vi "ingresaMediciones.vi"(8 "error in (no error)":errorcluster, 9 "Tbl Refnum":refnum<vi>, 10 "New Value":string[][](array[string]), 11 "Prueba06 in":refnum<class "Prueba06.lvclass">) -> (0 "error out":errorcluster, 3 "Prueba06 out":refnum<class "Prueba06.lvclass">)   [LabVIEW 2019, in "Prueba06.lvclass"]
uses:
  Prueba06.lvclass
  Prueba06.lvclass/Prueba06.ctl
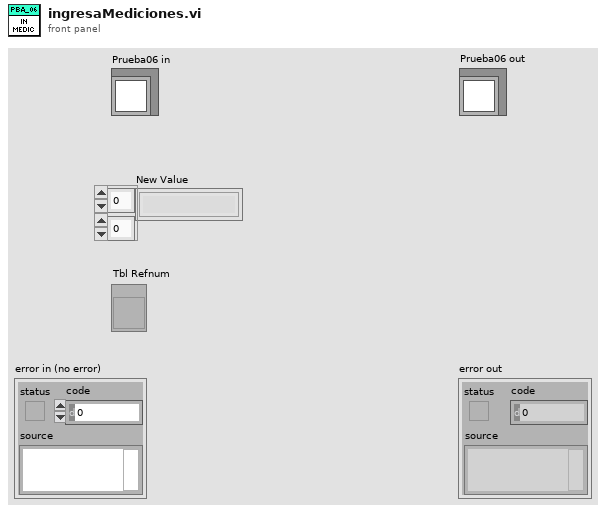
[diagram p1: front panel]
types:
  T1 = cluster{"Medido":dbl, "Error":dbl, "Ref":dbl, "Incert_exp":dbl, "Tol+":dbl, "Tol-":dbl, "fila":i32}
  T2 = typedef "LVRowAndColumnTypeDef.ctl" = cluster{"Row":i32, "Column":i32}
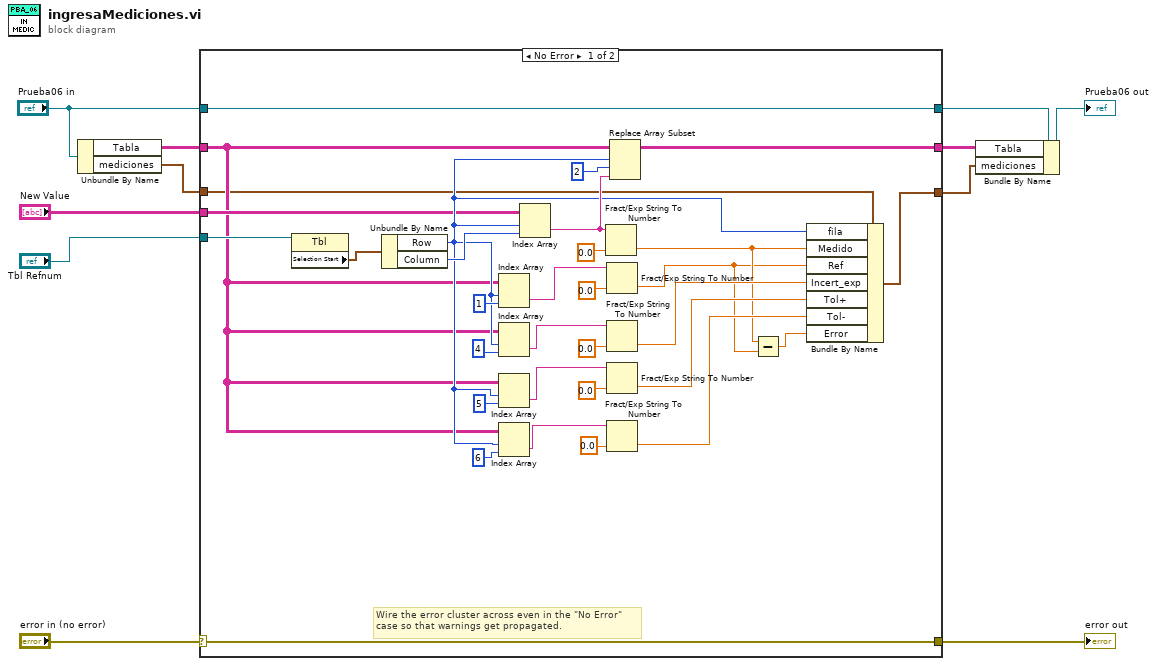
[diagram p0: block diagram]
diagram:
  n1 = Unbundle By Name("Prueba06 in") -> ("Tabla"=w5:string[][], "mediciones"=w4:T1)
  n2 = case shown="No Error" "error in (no error)" {
    selector: "error in (no error)" -> [w42 w47]
    tunnel: [w42 w47] -> w10
    tunnel: [w43 w46] -> w9
    tunnel: "Prueba06 in" -> [w43 w46]
    tunnel: w5 -> [w18 w45]
    tunnel: "New Value" -> [w21 _]
    tunnel: "Tbl Refnum" -> [w20 _]
    tunnel: w4 -> [w17 w44]
    tunnel: [w16 w45] -> w2
    tunnel: [w15 w44] -> w1
    frame No Error {
      # "Wire the error cluster across even in the \"No Error\"\ncase so that warnings get propagated."
      n3 = property on="Property Node" class="Tbl"(reference=w20) -> ("Selection Start"=w19:T2)  [unwired: 1 in, 2 out]
      n4 = Unbundle By Name(w19) -> ("Row"=w22:i32, "Column"=w39:i32)
      n5 = Index Array(array=w18, index (row)=w22, index (col)=1 ("disabled index (col)")) -> (element=w37:string)
      n6 = Index Array(array=w18, index (row)=w22, index (col)=4 ("index (row)")) -> (element=w33:string)
      n7 = Index Array(array=w18, index (row)=w22, index (col)=5 ("disabled index (col)")) -> (element=w24:string)
      n8 = Index Array(array=w18, index (row)=w22, index (col)=6 ("index (row)")) -> (element=w27:string)
      n9 = Index Array(array=w21, index (row)=w22, index (col)=w39) -> (element=w23:string)
      n10 = Fract/Exp String To Number(string=w23, default (0 dbl)=0.0) -> (number=w14:dbl)  [unwired: 2 in, 1 out]
      n11 = Fract/Exp String To Number(string=w37, default (0 dbl)=0.0) -> (number=w13:dbl)  [unwired: 2 in, 1 out]
      n12 = Fract/Exp String To Number(string=w33, default (0 dbl)=0.0) -> (number=w32:dbl)  [unwired: 2 in, 1 out]
      n13 = Fract/Exp String To Number(string=w24, default (0 dbl)=0.0) -> (number=w25:dbl)  [unwired: 2 in, 1 out]
      n14 = Fract/Exp String To Number(string=w27, default (0 dbl)=0.0) -> (number=w26:dbl)  [unwired: 2 in, 1 out]
      n15 = Replace Array Subset(array=w18, new element=w23, index (row)=w22, index (col)=2 ("disabled index (col)")) -> (w16:string[][])
      n16 = Subtract(x=w14, y=w13) -> (x-y=w12:dbl)
      n17 = Bundle By Name(cluster=w17, "fila"=w22, "Medido"=w14, "Ref"=w13, "Incert_exp"=w32, "Tol+"=w25, "Tol-"=w26, "Error"=w12) -> (w15:T1)
    }
    frame Error {
    }
  }
  "error out" <- w10
  n18 = Bundle By Name(cluster=w9, "Tabla"=w2, "mediciones"=w1) -> (→"Prueba06 out":refnum<class "Prueba06.lvclass">)
